vi "ID.vi"(11 "Entity in":refnum<class "Entity.lvclass">) -> (2 "ID":T1, 3 "Entity out":refnum<class "Entity.lvclass">)   [LabVIEW 2020, in "Conditum.lvlib" / "Entity.lvclass"]
uses:
  Entity.lvclass
  Columns/ID/ID.lvclass
  Entity ID.ctl
  Conditum.lvlib
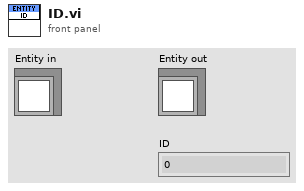
[diagram p1: front panel]
types:
  T1 = typedef "Conditum.lvlib/Entity ID.ctl" = i64
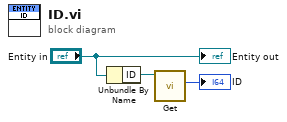
[diagram p0: block diagram]
diagram:
  n1 = Unbundle By Name("Entity in") -> ("ID"=w2:refnum<class "ID.lvclass">)
  n2 = call "Get.vi"("ID in"=w2) -> ("Entity ID"=→"ID":T1)  [unwired: 10 in]
  "Entity out" <- "Entity in"
